vi "Upd Full Scale Range.vi"(8 "error in (no error)":errorcluster, 10 "Full Scale Range":dbl, 11 "C100L in":refnum<class "C100L.lvclass">) -> (0 "error out":errorcluster, 3 "C100L out":refnum<class "C100L.lvclass">)   [LabVIEW 2021, in "C100L.lvlib" / "C100L.lvclass"]
uses:
  C100L.lvclass
  C100L.lvclass/C100L.ctl
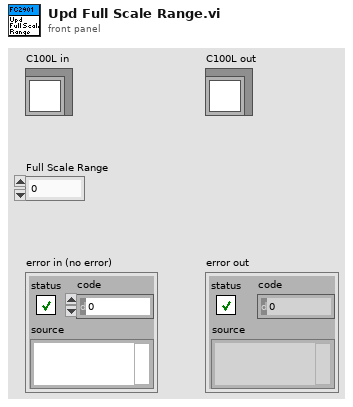
[diagram p1: front panel]
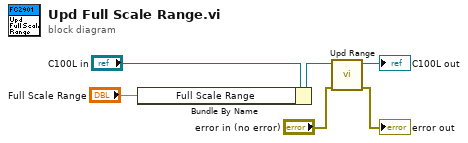
[diagram p0: block diagram]
diagram:
  n1 = Bundle By Name(cluster="C100L in", "Full Scale Range"="Full Scale Range") -> (w3:refnum<class "C100L.lvclass">)
  n2 = call "Upd Range.vi"("error in (no error)"="error in (no error)", "C100L in"=w3) -> ("error out"=→"error out":errorcluster, "C100L out"=→"C100L out":refnum<class "C100L.lvclass">)  [unwired: 8 in]
